vi "MessageName.vi"() -> (2 "MessageName":string)   [LabVIEW 2020, in "CmdAnalogMultiple.lvlib"]
uses:
  CmdAnalogMultiple.lvlib
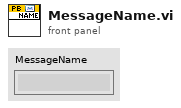
[diagram p1: front panel]
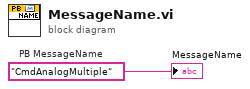
[diagram p0: block diagram]
diagram:
  w1 = "CmdAnalogMultiple"  # PB MessageName
  "MessageName" <- w1
